vi "Read ITC LPF Needle Valve.vi"(8 "error in (no error)":errorcluster, 11 "Instrument.Oxford1820 in":refnum<class "Instrument.OxfordVRM.lvclass">) -> (0 "error out":errorcluster, 2 "LPF Needle Valve (%)":dbl, 3 "Instrument.Oxford1820 out":refnum<class "Instrument.OxfordVRM.lvclass">)   [LabVIEW 2016, in "Instrument.OxfordVRM.lvclass"]
uses:
  Instrument.OxfordVRM.lvclass
  <instrlib>/Mercury iXX/Mercury iXX.lvlib
  <instrlib>/Mercury iXX/Public/Libraries/Auxiliary/Open/Open Auxiliary Device.vi
  <instrlib>/Mercury iXX/Public/Libraries/Auxiliary.lvlib
  <instrlib>/Mercury iXX/Public/Libraries/Auxiliary/Signals/Read/Percent Open (Read).vi
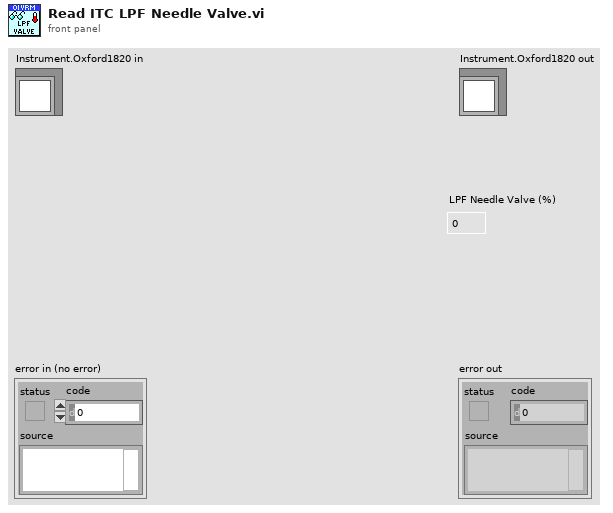
[diagram p1: front panel]
types:
  T1 = typedef "Mercury iXX.lvlib/Mercury Reference.ctl" = cluster{"Comms":refnum<visa-resource-name>, "Device ID":string[], "Comms Layer":T2, "Command":string, "Query reference":T3}
  T2 = typedef "Mercury iXX.lvlib/Comms Transport Layer.ctl" = enum16{"Ethernet TCP/IP", "USB", "ISOBus - RS-232", "GPIB"}
  T3 = typedef "Mercury iXX.lvlib/Query Dynamic Reference.ctl" = refnum<vi>
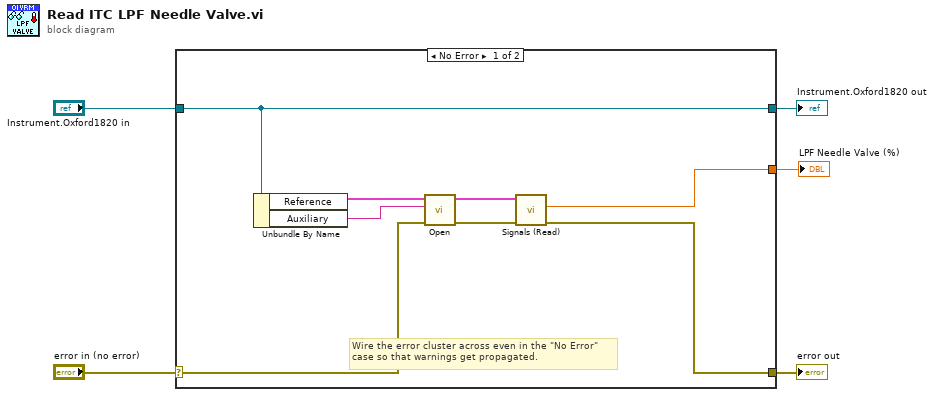
[diagram p0: block diagram]
diagram:
  n1 = case shown="No Error" "error in (no error)" {
    selector: "error in (no error)" -> [w10 w15]
    tunnel: [w7 w15] -> w4
    tunnel: [w13 w14] -> w2
    tunnel: "Instrument.Oxford1820 in" -> [w13 w14]
    tunnel: [w6 _] -> w1
    frame No Error {
      # "Wire the error cluster across even in the \"No Error\"\ncase so that warnings get propagated."
      n2 = Unbundle By Name(w13) -> ("Reference"=w12:T1, "Auxiliary"=w11:string)
      n3 = call-poly <instrlib>:"Open.vi"("error in (no error)"=w10, "Device Identifier"=w11, "Mercury Reference In"=w12) -> ("error out"=w8:errorcluster, "Mercury Reference Out"=w9:T1)  [unwired: 7 out]
      n4 = call-poly <instrlib>:"Signals (Read).vi"("error in"=w8, "Mercury Reference In"=w9) -> ("error out"=w7:errorcluster, "% Open"=w6:dbl)  [unwired: 1 in, 7 out]
    }
    frame Error {
    }
  }
  "error out" <- w4
  "Instrument.Oxford1820 out" <- w2
  "LPF Needle Valve (%)" <- w1
